vi "_attribute_read_int64.vi"(5 "Repeated Capability":string, 7 "Attribute":T1={"Identifier"="", "Descriptive Name"="", "Data Type"=enum."Integer 32", "Command"="", "Access"=enum."Read/Write", "Range Table"="", "Read Callback"="", "Write Callback"="", "Supported Models"="", "Instrument Options"="", "Index"=0, "OPC Wait"=FALSE, "No Status Check"=FALSE, "Cache Only"=FALSE}, 8 "error in":errorcluster caption="error in (no error)", 10 "Query Parameter":string, 11 "VISA resource name":refnum<visa-resource-name>) -> (0 "error out":errorcluster, 2 "Int64 out":i64, 3 "VISA resource name out":refnum<visa-resource-name>)   [LabVIEW 2022 SP3, in "hmp4000_rsidr_core.lvlib"]
uses:
  hmp4000_rsidr_core.lvlib
  type_Attribute.ctl
  type_Attribute_Data_Type.ctl
  type_ReadWriteAccess.ctl
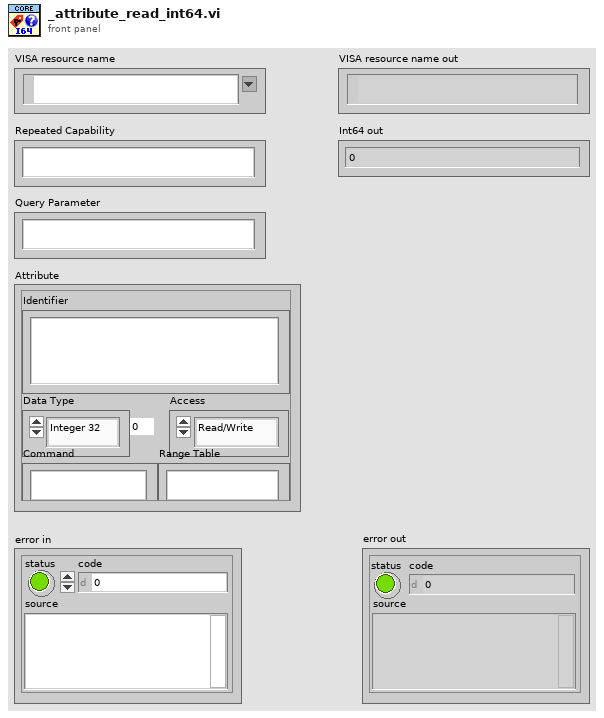
[diagram p1: front panel]
types:
  T1 = typedef "hmp4000_rsidr_core.lvlib/type_Attribute.ctl" = cluster{"Identifier":string, "Descriptive Name":string, "Data Type":T2, "Command":string, "Access":T3, "Range Table":string, "Read Callback":string, "Write Callback":string, "Supported Models":string, "Instrument Options":string, "Index":i32, "OPC Wait":bool, "No Status Check":bool, "Cache Only":bool}
  T2 = typedef "hmp4000_rsidr_core.lvlib/type_Attribute_Data_Type.ctl" = enum16{"Integer 32", "Double", "String", "Boolean", "None", "Integer 64", "RawString"}
  T3 = typedef "hmp4000_rsidr_core.lvlib/type_ReadWriteAccess.ctl" = enum16{"Read Only", "Write Only", "Read/Write"}
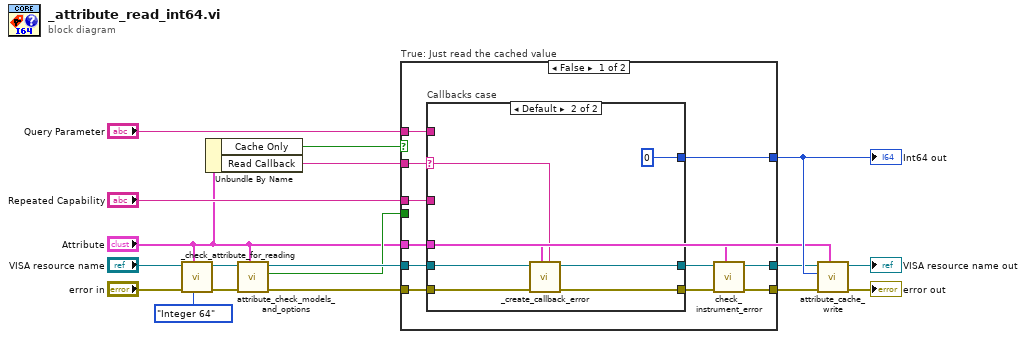
[diagram p0: block diagram]
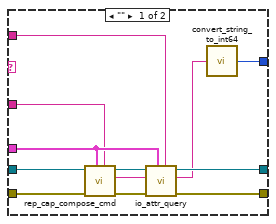
[diagram p2: hidden frame]
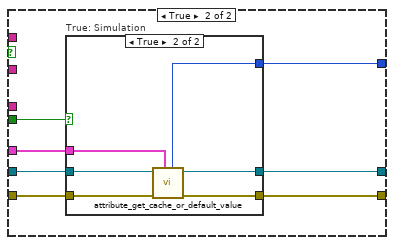
[diagram p3: hidden frame]
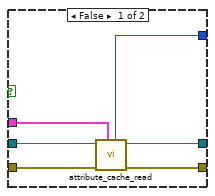
[diagram p4: hidden frame]
diagram:
  n1 = call "_check_attribute_for_reading.vi"("Expected Data Type"=type_Attribute_Data_Type."Integer 64" ("Data Type"), "Attribute"="Attribute", "error in"="error in", "VISA resource name"="VISA resource name") -> ("error out"=w9:errorcluster, "VISA resource name out"=w8:refnum<visa-resource-name>)  [unwired: 6 in]
  n2 = Unbundle By Name("Attribute") -> ("Cache Only"=w1:bool, "Read Callback"=w10:string)
  n3 = call "attribute_check_models_and_options.vi"("Attribute"="Attribute", "error in"=w9, "VISA resource name"=w8) -> ("error out"=w7:errorcluster, "Simulation Mode"=w5:bool, "VISA resource name out"=w6:refnum<visa-resource-name>)  [unwired: 6 in]
  n4 = case "True: Just read the cached value" shown="False" w1 {
    tunnel: "Repeated Capability" -> [w29 _]
    tunnel: [w21 w53] -> w4
    tunnel: [w20 w52] -> w3
    tunnel: [w28 w50] -> w13
    tunnel: w10 -> [w27 _]
    tunnel: w6 -> [w26 w55]
    tunnel: w7 -> [w25 w54]
    tunnel: "Attribute" -> [w19 w51]
    tunnel: w5 -> [_ w49]
    tunnel: "Query Parameter" -> [w24 _]
    frame False {
      n5 = case "Callbacks case" shown="Default" w27 {
        selector: w27 -> [_ w42]
        tunnel: w26 -> [w41 w46]
        tunnel: w25 -> [w40 w47]
        tunnel: w29 -> [w34 _]
        tunnel: [w33 w44] -> w22
        tunnel: [w31 w45] -> w23
        tunnel: [w39 i64 0 ("int64 value out")] -> w28
        tunnel: w19 -> [w35 w43]
        tunnel: w24 -> [w30 _]
        frame "" {
          n6 = call "rep_cap_compose_cmd.vi"("Repeated Capability"=w34, "Attribute"=w35, "error in"=w40, "VISA resource name"=w41) -> ("error out"=w38:errorcluster, "Command out"=w36:string, "VISA resource name out"=w37:refnum<visa-resource-name>)  [unwired: 5 in]
          n7 = call "io_attr_query.vi"("Query Parameter (None)"=w30, "Attribute"=w35, "error in"=w38, "write buffer"=w36, "VISA resource name"=w37) -> ("error out"=w31:errorcluster, "read buffer"=w32:string, "VISA resource name out"=w33:refnum<visa-resource-name>)  [unwired: 4 in]
          n8 = call "convert_string_to_int64.vi"("String in"=w32) -> ("int64 value out"=w39:i64)  [unwired: 4 in]
        }
        frame Default {
          n9 = call "_create_callback_error.vi"("Callback Name"=w42, "Attribute"=w43, "error in"=w47, "VISA resource name"=w46) -> ("error out"=w45:errorcluster, "VISA resource name out"=w44:refnum<visa-resource-name>)  [unwired: 6 in]
        }
      }
      n10 = call "check_instrument_error.vi"("Attribute"=w19, "error in"=w23, "VISA resource name"=w22) -> ("error out"=w21:errorcluster, "VISA resource name out"=w20:refnum<visa-resource-name>)  [unwired: 7 in]
    }
    frame True {
      n11 = case "True: Simulation" shown="True" w49 {
        tunnel: w54 -> [w61 w67]
        tunnel: w55 -> [w60 w66]
        tunnel: w51 -> [w59 w63]
        tunnel: [w58 w65] -> w53
        tunnel: [w57 w64] -> w52
        tunnel: [w56 w62] -> w50
        frame False {
          n12 = call "attribute_cache_read.vi"("Attribute"=w59, "error in"=w61, "VISA resource name"=w60) -> ("error out"=w58:errorcluster, "VISA resource name out"=w57:refnum<visa-resource-name>, "Int64 out"=w56:i64)  [unwired: 1 in, 5 out]
        }
        frame True {
          n13 = call "attribute_get_cache_or_default_value.vi"("Attribute"=w63, "error in"=w67, "VISA resource name"=w66) -> ("error out"=w65:errorcluster, "VISA resource name out"=w64:refnum<visa-resource-name>, "Int64 out"=w62:i64)  [unwired: 1 in, 5 out]
        }
      }
    }
  }
  "Int64 out" <- w13
  n14 = call "attribute_cache_write.vi"("Attribute"="Attribute", "error in"=w4, "Value in"=w13, "VISA resource name"=w3) -> ("error out"=→"error out":errorcluster, "VISA resource name out"=→"VISA resource name out":refnum<visa-resource-name>)  [unwired: 6 in]
